vi "DrawEllipseCenter.vi"(8 "error in":errorcluster, 10 "Ellipse":T1 {"Minor Axis"."Point 2"."Y" format="%.2f"; "Minor Axis"."Point 2"."X" format="%.2f"; "Minor Axis"."Point 1"."Y" format="%.2f"; "Minor Axis"."Point 1"."X" format="%.2f"; "Major Axis"."Point 2"."Y" format="%.2f"; "Major Axis"."Point 2"."X" format="%.2f"; "Major Axis"."Point 1"."Y" format="%.2f"; "Major Axis"."Point 1"."X" format="%.2f"; "Center"."Y" format="%.2f"; "Center"."X" format="%.2f"}, 11 "Image in":T2) -> (0 "error out":errorcluster, 3 "Image out":T2)   [LabVIEW 2014]
uses:
  <vilib>/vision/Image Controls.llb/IMAQ Image.ctl
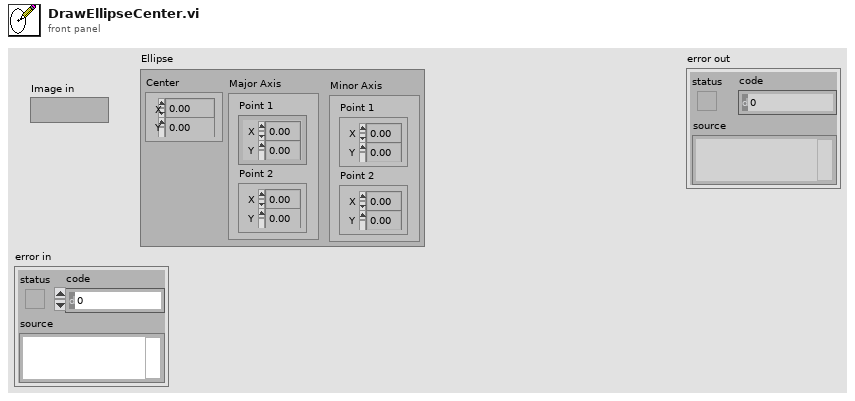
[diagram p1: front panel]
types:
  T1 = cluster{"Center":cluster{"X":sgl, "Y":sgl}, "Major Axis":cluster{"Point 1":cluster{"X":sgl, "Y":sgl}, "Point 2":cluster{"X":sgl, "Y":sgl}}, "Minor Axis":cluster{"Point 1":cluster{"X":sgl, "Y":sgl}, "Point 2":cluster{"X":sgl, "Y":sgl}}}
  T2 = typedef "IMAQ Image.ctl" = refnum<image>
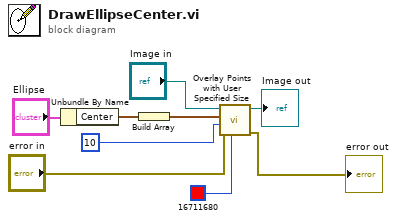
[diagram p0: block diagram]
diagram:
  n1 = Unbundle By Name("Ellipse") -> ("Center"=w3:cluster{"X":sgl, "Y":sgl})
  n2 = Build Array(w3) -> (w8:cluster{"X":sgl, "Y":sgl}[])
  n3 = call "Overlay Points with User Specified Size.vi"("Color"=u32 16711680, "error in"="error in", "Point Diameter (5)"=u32 10, "Points"=w8, "Image In"="Image in") -> ("error out"=→"error out":errorcluster, "Image Out"=→"Image out":T2)  [unwired: 5 in]
